vi "Build State Subcase.vi"(8 "error in":errorcluster, 9 "State subcase":string, 11 "Parent State":string) -> (0 "error out":errorcluster, 3 "State out":string)   [LabVIEW 2013, in "State Machine Lib.lvlib"]
doc: "Takes 2 state strings and builds a new hierarchial state Parent State:Substate"
uses:
  State Machine Lib.lvlib
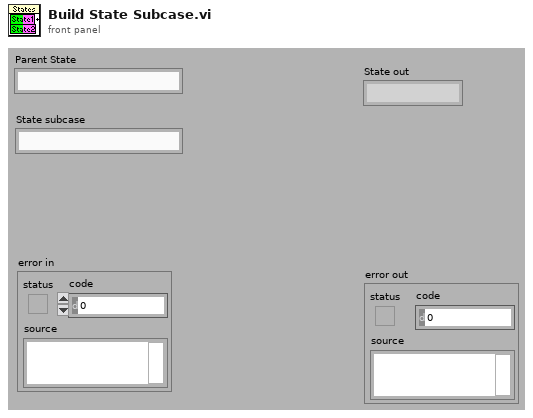
[diagram p1: front panel]
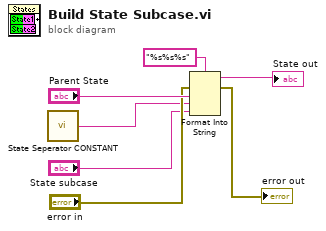
[diagram p0: block diagram]
diagram:
  n1 = call "State Seperator CONSTANT.vi"() -> ("Seperator (:)"=w1:string)
  n2 = Format Into String(format string="%s%s%s" ("regular expression"), error in="error in", "Parent State", w1, "State subcase") -> (resulting string=→"State out":string, error out=→"error out":errorcluster)  [unwired: 1 in]
